vi "comm timeout2.vi"(5 "ulReadIntervalTimeout":u32, 6 "ulWriteTotalTimeoutMultiplier":u32, 7 "ulReadTotalTimeoutMultiplier":u32, 8 "error in (no error)":errorcluster, 9 "ulWriteTotalTimeoutConstant":u32, 10 "ulReadTotalTimeoutConstant":u32, 11 "Comm Handle":u64) -> (0 "error out":errorcluster, 3 "dup Comm Handle":u64)   [LabVIEW 2009, in "lvserial.lvlib"]
doc: "Configures the timeout value for read and write operations."
uses:
  lvserial.lvlib
  x64/Release/lvserial.dll
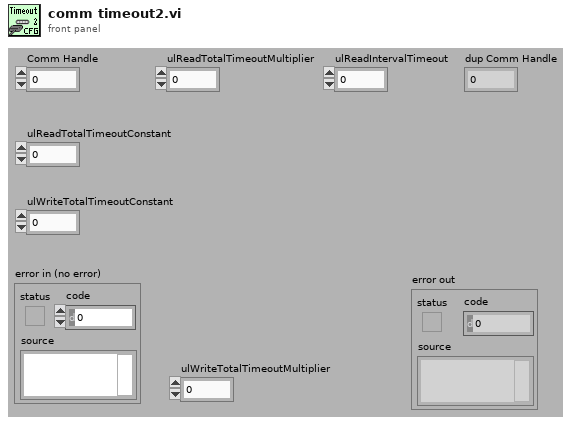
[diagram p1: front panel]
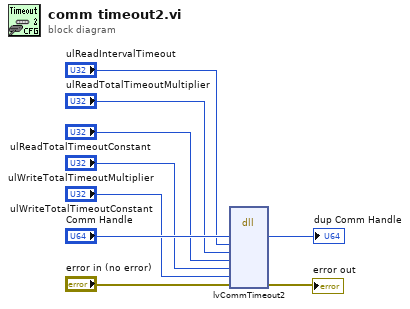
[diagram p0: block diagram]
diagram:
  n1 = dll-call lib="C:/Users/Admin/Desktop/lvserial_source_1-2-13/x64/Release/lvserial.dll" fn="lvCommTimeout2"("hComm"="Comm Handle", "ulReadIntervalTimeout"="ulReadIntervalTimeout", "ulReadTotalTimeoutMultiplier"="ulReadTotalTimeoutMultiplier", "ulReadTotalTimeoutConstant"="ulReadTotalTimeoutConstant", "ulWriteTotalTimeoutMultiplier"="ulWriteTotalTimeoutMultiplier", "ulWriteTotalTimeoutConstant"="ulWriteTotalTimeoutConstant", "error"="error in (no error)") -> ("hComm"=→"dup Comm Handle":u64, "error"=→"error out":errorcluster)  [unwired: 8 in, 3 out]
